vi "Calculate MD5 for Configuration File.vi"(8 "error in (no error)":errorcluster, 10 "runtime? (F)":bool, 11 "Item Ref in":T1 format="%.0x") -> (0 "error out":errorcluster, 2 "MD5":string, 3 "Device Ref out":T1 format="%.0x")   [LabVIEW 2017, in "DSF Shared.lvlib"]
uses:
  Shared/DSF Shared.lvlib
  <vilib>/NI Veristand/Custom Device API/Custom Device Item Ref.ctl
  DSF System Explorer.lvlib
  <vilib>/NI Veristand/Custom Device API/Custom Device API.lvlib
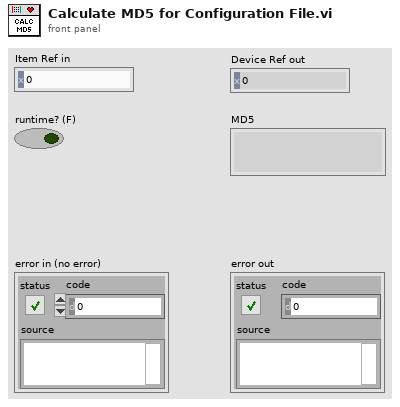
[diagram p1: front panel]
types:
  T1 = typedef "Custom Device API.lvlib/Custom Device Item Ref.ctl" = u64
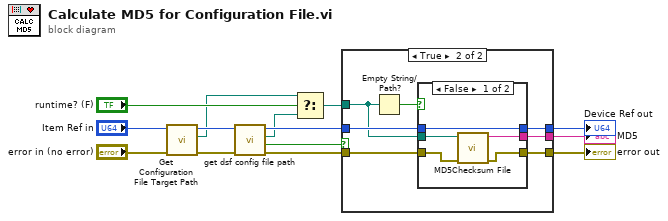
[diagram p0: block diagram]
diagram:
  n1 = call "Get Configuration File Target Path.vi"("error in (no error)"="error in (no error)", "Item Ref in"="Item Ref in") -> ("error out"=w5:errorcluster, "configuration target path"=w3:path, "Item Ref out"=w6:T1)  [unwired: 7 in]
  n2 = call "get dsf config file path.vi"("error in (no error)"=w5, "Node Ptr"=w6) -> ("error out"=w14:errorcluster, "Found?"=w13:bool, "Path"=w2:path, "Item Ref out"=w11:T1)  [unwired: 6 in]
  n3 = Select(t=w3, s="runtime? (F)", f=w2) -> (s? t:f=w1:path)
  n4 = case shown="True" w13 {
    tunnel: w14 -> [w16 w23]
    tunnel: w1 -> [_ w19]
    tunnel: [w16 w21] -> w12
    tunnel: w11 -> [w15 w22]
    tunnel: [w15 w20] -> w10
    tunnel: [_ w17] -> w9
    frame False {
    }
    frame True {
      n5 = Empty String/Path?(string/path=w19) -> (empty?=w18:bool)
      n6 = case shown="False" w18 {
        tunnel: w23 -> [w28 w30]
        tunnel: w22 -> [w27 w29]
        tunnel: [w26 w30] -> w21
        tunnel: [w27 w29] -> w20
        tunnel: w19 -> [w25 _]
        tunnel: [w24 _] -> w17
        frame False {
          n7 = call <vilib>:"MD5Checksum File.vi"("error in (no error)"=w28, "Path"=w25) -> ("error out"=w26:errorcluster, "MD5 message-digest"=w24:string)  [unwired: 8 in]
        }
        frame True {
        }
      }
    }
  }
  "Device Ref out" <- w10
  "error out" <- w12
  "MD5" <- w9
